vi "rrQA_Sub3.vi"(0 "U":dbl[](array[numeric]) format="%.2f", 2 "W":dbl[](array[numeric]) format="%.2f", 3 "T":dbl[](array[numeric]) format="%.2f") -> ()   [LabVIEW 2010]
uses:
  <vilib>/Utility/file.llb/Write To Spreadsheet File (DBL).vi
  <vilib>/Analysis/NI_AALBase.lvlib
panel:
  in  "u', w' data file":path
  out "Mean Time between events":dbl[](array[numeric])
  out "Loop Frame 1":i32
  out "Loop Frame 0":i32
  in  "LDA data?":bool
  in  "QA results file":path
  out "Quadrant shear totals":dbl[](array[numeric]) format="%.3f"
  out "% Time Spent in Quadrant":dbl[](array[numeric])
  out "u'w' (bar) total":dbl format="%.3f"
  in  "Threshold Array, H":dbl[](array[numeric])=[0.1] format="%.2f"
  out "XY Graph":cluster{dbl[], dbl[]}(graph)
  # "Quadrant Analysis Subroutine for Two-Component Velocity Data"
  # "Version 2.1 -RR"
  # "- FOR MANUAL ENTRY -"
  # "- ANALYSIS (OUTPUT) -"
  # "- FILE TO CREATE -"
  # "- THRESHOLD ARRAY -"
  # "- FOR PLUG-IN USE -"
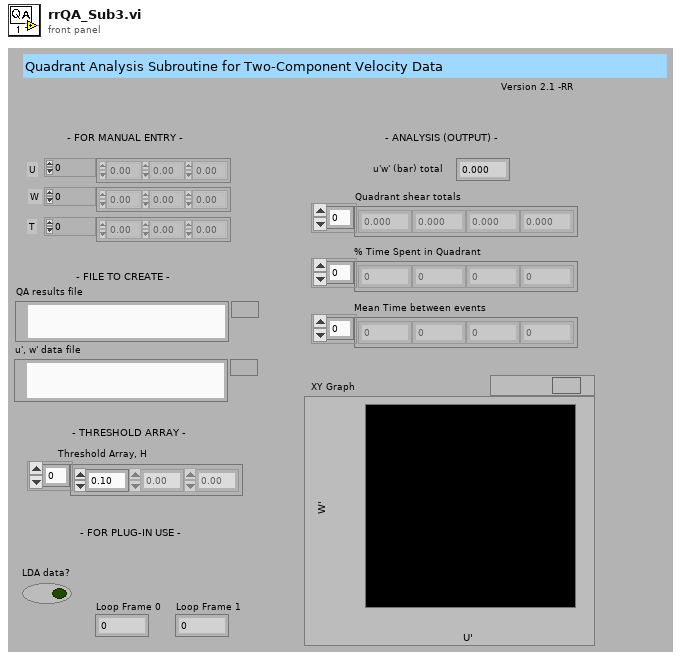
[diagram p1: front panel]
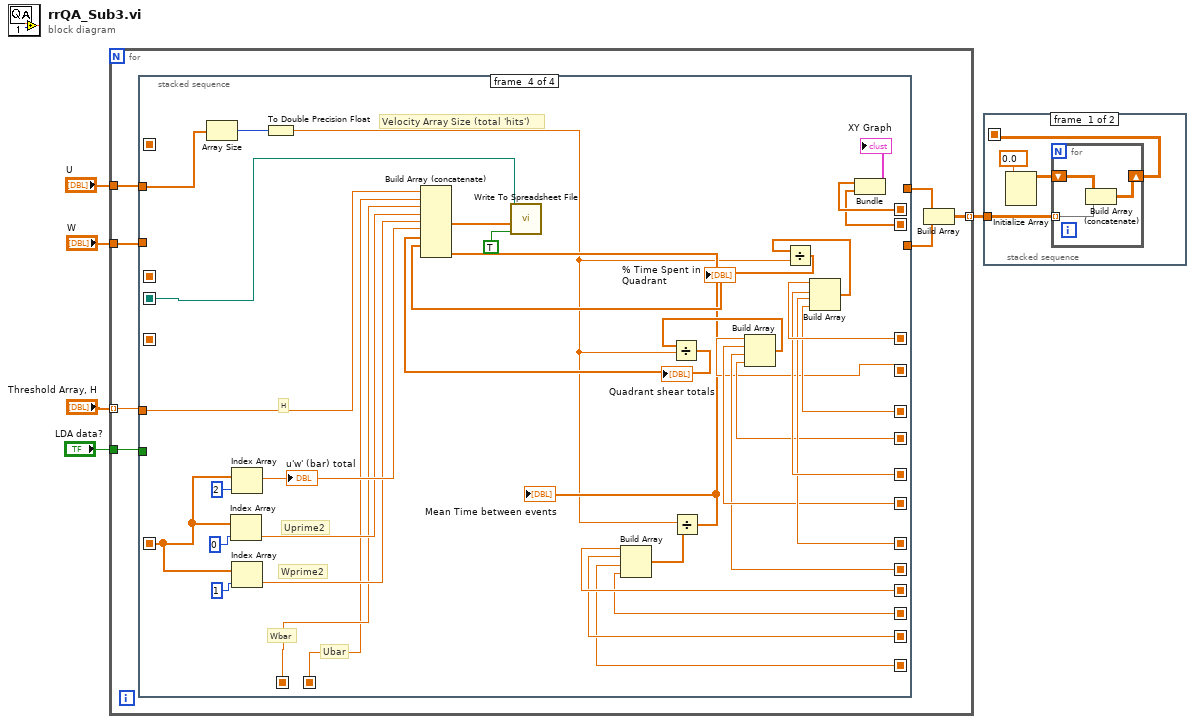
[diagram p0: block diagram]
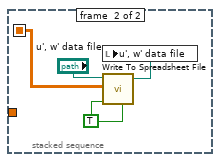
[diagram p2: hidden frame]
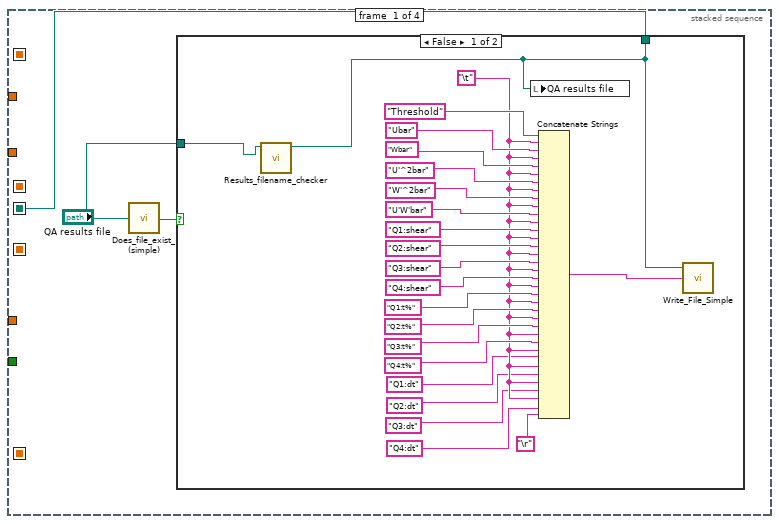
[diagram p3: hidden frame]
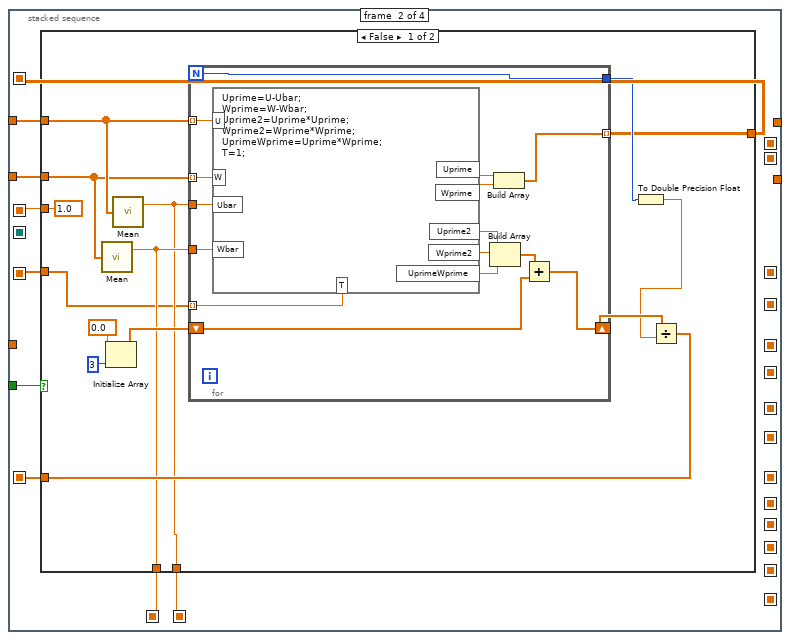
[diagram p5: hidden frame]
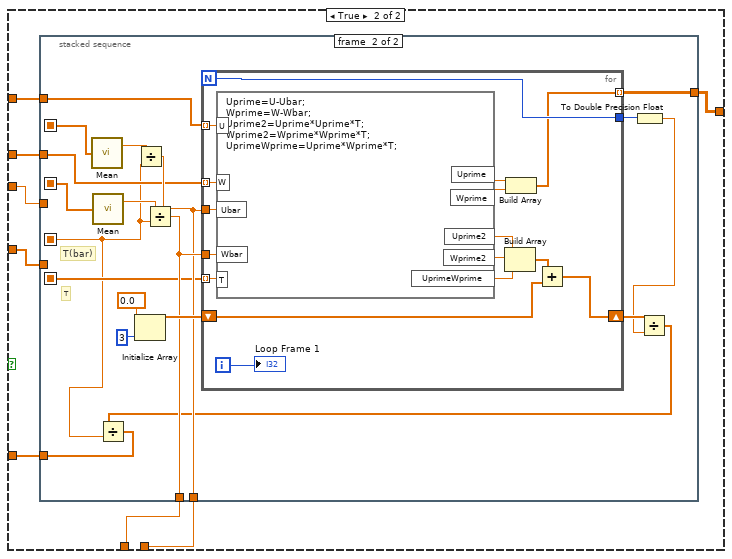
[diagram p6: hidden frame]
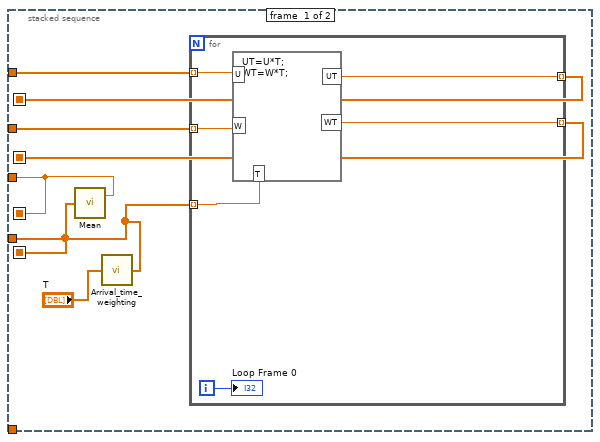
[diagram p7: hidden frame]
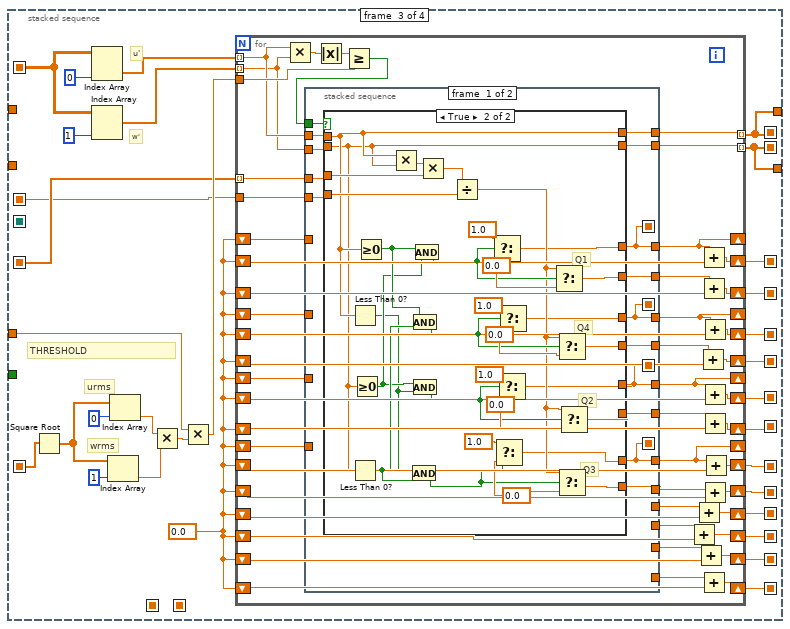
[diagram p8: hidden frame]
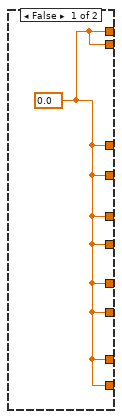
[diagram p9: hidden frame]
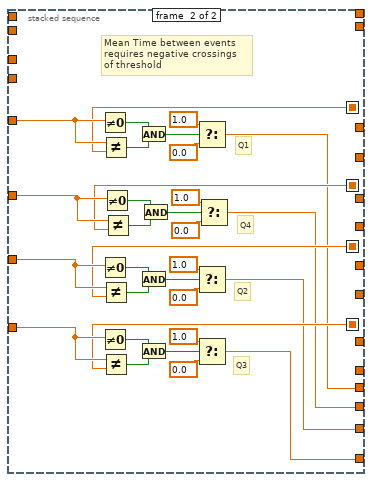
[diagram p10: hidden frame]
diagram:
  n1 = for {
    tunnel: "Threshold Array, H" -> [w12] mode=indexing
    tunnel: "U" -> [w11]
    tunnel: "W" -> [w10]
    tunnel: "LDA data?" -> [w9]
    tunnel: [w6] -> w1 mode=indexing
    n2 = stacked-sequence {
      seq-local: [_ w48 _ _] -> [_ _ w145 w319]
      seq-local: [_ _ w152 _] -> [_ _ _ w306]
      seq-local: [_ _ w153 _] -> [_ _ _ w329]
      seq-local: [_ _ w151 _] -> [_ _ _ w326]
      seq-local: [_ _ w150 _] -> [_ _ _ w322]
      seq-local: [_ _ w149 _] -> [_ _ _ w328]
      seq-local: [_ _ w148 _] -> [_ _ _ w324]
      seq-local: [_ _ w147 _] -> [_ _ _ w327]
      seq-local: [_ _ w146 _] -> [_ _ _ w323]
      seq-local: [_ w46 _ _] -> [_ _ _ w305]
      seq-local: [_ w45 _ _] -> [_ _ _ w304]
      seq-local: [_ w44 _ _] -> [_ _ w143 _]
      seq-local: [_ w43 _ _] -> [_ _ w144 _]
      seq-local: [_ w42 _ _] -> [_ _ w142 _]
      seq-local: [w15 _ _ _] -> [_ _ _ w314]
      seq-local: [_ _ w134 _] -> [_ _ _ w294]
      seq-local: [_ _ w135 _] -> [_ _ _ w295]
      seq-local: [_ _ w140 _] -> [_ _ _ w303]
      seq-local: [_ _ w139 _] -> [_ _ _ w302]
      seq-local: [_ _ w138 _] -> [_ _ _ w301]
      seq-local: [_ _ w137 _] -> [_ _ _ w300]
      tunnel: w9 -> [_ w47 _ _]
      tunnel: w11 -> [_ w41 _ w313]
      tunnel: w10 -> [_ w40 _ _]
      tunnel: w12 -> [_ _ w141 w296]
      tunnel: [_ _ w135 _] -> w8
      tunnel: [_ _ w134 _] -> w7
      frame #0 {
        n3 = call "Does_file_exist_(simple).vi"("Pathname"="QA results file") -> ("exists?"=w13:bool)
        n4 = case shown="False" w13 {
          tunnel: [w16 w39] -> w15
          tunnel: "QA results file" -> [w17 w39]
          frame False {
            w22 = "\t"
            n5 = call "Results_filename_checker.vi"("Results file"=w17) -> ("Results file output"=w16:path)  [unwired: 4 in, 3 out]
            n6 = local write "QA results file"(w16) -> ()
            n7 = Concatenate Strings("Threshold", w22, "Ubar", w22, "Wbar", w22, "U'^2bar", w22, "W'^2bar", w22, "U'W'bar", w22, "Q1:shear", w22, "Q2:shear", w22, "Q3:shear", w22, "Q4:shear", w22, "Q1:t%", w22, "Q2:t%", w22, "Q3:t%", w22, "Q4:t%", w22, "Q1:dt", w22, "Q2:dt", w22, "Q3:dt", w22, "Q4:dt", "\r") -> (w27:string)
            n8 = call "Write_File_Simple.vi"("character string"=w27, "file path"=w16) -> ()  [unwired: 1 in, 2 out]
          }
          frame True {
          }
        }
      }
      frame #1 {
        n9 = case shown="False" w47 {
          tunnel: [w58 w81] -> w48
          tunnel: w41 -> [w55 w85]
          tunnel: w40 -> [w54 w84]
          tunnel: [w53 w83] -> w46
          tunnel: [w52 w82] -> w45
          tunnel: [1.0 w80] -> w44
          tunnel: [w50 w79] -> w43
          tunnel: [w49 w78] -> w42
          frame False {
            n10 = call <vilib>:"Mean.vi"("X"=w54) -> ("mean"=w53:dbl)  [unwired: 1 out]
            n11 = Initialize Array(0.0, 3) -> (w61:dbl[])
            n12 = call <vilib>:"Mean.vi"("X"=w55) -> ("mean"=w52:dbl)  [unwired: 1 out]
            n13 = for {
              N -> [w68]
              tunnel: w55 -> [w77] mode=indexing
              tunnel: w54 -> [w76] mode=indexing
              shift-right: [w69] -> w59
              shift-left: w61 -> [w70]
              tunnel: [w68] -> w57
              tunnel: w52 -> [w66]
              tunnel: w53 -> [w65]
              tunnel: [w64] -> w50 mode=indexing
              tunnel: [w63] -> w49 mode=indexing
              n14 = formula code="Uprime=U-Ubar;\nWprime=W-Wbar;\nUprime2=Uprime*Uprime;\nWprime2=Wprime*Wprime;\nUprimeWprime=Uprime*Wprime;\nT=1;"("W"=w76, "U"=w77, "Ubar"=w66, "Wbar"=w65) -> ("Uprime"=w75:dbl, "Wprime"=w74:dbl, "Uprime2"=w73:dbl, "Wprime2"=w72:dbl, "UprimeWprime"=w67:dbl, "T"=w64:dbl)
              n15 = Build Array(w73, w72, w67) -> (w71:dbl[])
              n16 = Build Array(w75, w74) -> (w63:dbl[])
              n17 = Add(x=w71, y=w70) -> (x+y=w69:dbl[])
            }
            n18 = To Double Precision Float(number=w57) -> (double precision float=w56:dbl)
            n19 = Divide(x=w59, y=w56) -> (x/y=w58:dbl[])
          }
          frame True {
            n20 = stacked-sequence {
              seq-local: [w90 _] -> [_ w113]
              seq-local: [w89 _] -> [_ w114]
              seq-local: [w88 _] -> [_ w102]
              seq-local: [w86 _] -> [_ w106]
              tunnel: w85 -> [w92 w108]
              tunnel: w84 -> [w91 w107]
              tunnel: [_ w112] -> w83
              tunnel: [_ w109] -> w82
              tunnel: [_ w101] -> w81
              tunnel: [w88 _] -> w80
              tunnel: [w86 _] -> w79
              tunnel: [_ w99] -> w78
              frame #0 {
                n21 = call "Arrival_time_weighting.vi"("Arrival times"="T") -> ("Weighting"=w86:dbl[])
                n22 = call <vilib>:"Mean.vi"("X"=w86) -> ("mean"=w88:dbl)  [unwired: 1 out]
                n23 = for {
                  tunnel: w92 -> [w98] mode=indexing
                  tunnel: w91 -> [w97] mode=indexing
                  tunnel: w86 -> [w96] mode=indexing
                  tunnel: [w95] -> w90 mode=indexing
                  tunnel: [w94] -> w89 mode=indexing
                  i -> [w93]
                  n24 = formula code="UT=U*T;\nWT=W*T;"("T"=w96, "U"=w98, "W"=w97) -> ("UT"=w95:dbl, "WT"=w94:dbl)
                  "Loop Frame 0" <- w93
                }
              }
              frame #1 {
                # "T"
                # "T(bar)"
                n25 = call <vilib>:"Mean.vi"("X"=w113) -> ("mean"=w111:dbl)  [unwired: 1 out]
                n26 = call <vilib>:"Mean.vi"("X"=w114) -> ("mean"=w110:dbl)  [unwired: 1 out]
                n27 = Initialize Array(0.0, 3) -> (w115:dbl[])
                n28 = Divide(x=w111, y=w102) -> (x/y=w109:dbl)
                n29 = Divide(x=w110, y=w102) -> (x/y=w112:dbl)
                n30 = for {
                  N -> [w124]
                  tunnel: w108 -> [w133] mode=indexing
                  tunnel: w107 -> [w132] mode=indexing
                  shift-right: [w125] -> w104
                  shift-left: w115 -> [w126]
                  tunnel: [w124] -> w105
                  tunnel: w109 -> [w122]
                  tunnel: w112 -> [w121]
                  tunnel: w106 -> [w120] mode=indexing
                  tunnel: [w119] -> w99 mode=indexing
                  i -> [w118]
                  n31 = formula code="Uprime=U-Ubar;\nWprime=W-Wbar;\nUprime2=Uprime*Uprime*T;\nWprime2=Wprime*Wprime*T;\nUprimeWprime=Uprime*Wprime*T;"("W"=w132, "U"=w133, "Ubar"=w122, "Wbar"=w121, "T"=w120) -> ("Uprime"=w131:dbl, "Wprime"=w130:dbl, "Uprime2"=w129:dbl, "Wprime2"=w128:dbl, "UprimeWprime"=w123:dbl)
                  n32 = Build Array(w129, w128, w123) -> (w127:dbl[])
                  n33 = Build Array(w131, w130) -> (w119:dbl[])
                  n34 = Add(x=w127, y=w126) -> (x+y=w125:dbl[])
                  "Loop Frame 1" <- w118
                }
                n35 = To Double Precision Float(number=w105) -> (double precision float=w103:dbl)
                n36 = Divide(x=w104, y=w103) -> (x/y=w100:dbl[])
                n37 = Divide(x=w100, y=w102) -> (x/y=w101:dbl[])
              }
            }
          }
        }
      }
      frame #2 {
        w136 = 0.0
        # "THRESHOLD"
        # "wrms"
        # "urms"
        # "w'"
        # "u'"
        n38 = Square Root(x=w145) -> (sqrt(x)=w162:dbl[])
        n39 = Index Array(array=w142, index (col)=0) -> (element=w156:dbl[])  [unwired: 1 in]
        n40 = Index Array(array=w142, index (col)=1) -> (element=w155:dbl[])  [unwired: 1 in]
        n41 = Index Array(array=w162, index=1) -> (element=w158:dbl)
        n42 = Index Array(array=w162, index=0) -> (element=w159:dbl)
        n43 = Multiply(x=w159, y=w158) -> (x*y=w157:dbl)
        n44 = Multiply(x=w141, y=w157) -> (x*y=w154:dbl)
        n45 = for {
          tunnel: w156 -> [w202] mode=indexing
          tunnel: w155 -> [w201] mode=indexing
          tunnel: w154 -> [w212]
          tunnel: [w200] -> w135 mode=indexing
          tunnel: [w199] -> w134 mode=indexing
          shift-right: [w208] -> w152
          shift-left: w136 -> [w191]
          shift-right: [w211] -> w150
          shift-left: w136 -> [w189]
          shift-right: [w210] -> w148
          shift-left: w136 -> [w187]
          shift-right: [w209] -> w146
          shift-left: w136 -> [w185]
          shift-right: [w204] -> w153
          shift-left: w136 -> [w192]
          shift-right: [w207] -> w151
          shift-left: w136 -> [w190]
          shift-right: [w206] -> w149
          shift-left: w136 -> [w188]
          shift-right: [w205] -> w147
          shift-left: w136 -> [w186]
          tunnel: w144 -> [w198] mode=indexing
          tunnel: w143 -> [w197]
          shift-right: [w184] -> _
          shift-left: w136 -> [w180]
          shift-right: [w183] -> _
          shift-left: w136 -> [w177]
          shift-right: [w182] -> _
          shift-left: w136 -> [w178]
          shift-right: [w181] -> _
          shift-left: w136 -> [w179]
          shift-right: [w172] -> w140
          shift-left: w136 -> [w168]
          shift-right: [w171] -> w139
          shift-left: w136 -> [w167]
          shift-right: [w170] -> w138
          shift-left: w136 -> [w166]
          shift-right: [w169] -> w137
          shift-left: w136 -> [w165]
          n46 = Multiply(x=w202, y=w201) -> (x*y=w214:dbl)
          n47 = Absolute Value(x=w214) -> (abs(x)=w213:dbl)
          n48 = Greater Or Equal?(x=w213, y=w212) -> (x >= y?=w203:bool)
          n49 = stacked-sequence {
            seq-local: [w218 _] -> [_ w269]
            seq-local: [w217 _] -> [_ w268]
            seq-local: [w216 _] -> [_ w267]
            seq-local: [w215 _] -> [_ w266]
            tunnel: w203 -> [w229 _]
            tunnel: w202 -> [w228 _]
            tunnel: w201 -> [w227 _]
            tunnel: [w226 _] -> w200
            tunnel: [w225 _] -> w199
            tunnel: w198 -> [w224 _]
            tunnel: w197 -> [w223 _]
            tunnel: [w218 _] -> w184
            tunnel: [w222 _] -> w196
            tunnel: [w217 _] -> w183
            tunnel: [w221 _] -> w195
            tunnel: [w216 _] -> w182
            tunnel: [w220 _] -> w194
            tunnel: [w215 _] -> w181
            tunnel: [w219 _] -> w193
            tunnel: w180 -> [_ w270]
            tunnel: w179 -> [_ w273]
            tunnel: w178 -> [_ w272]
            tunnel: w177 -> [_ w271]
            tunnel: [_ w265] -> w176
            tunnel: [_ w264] -> w175
            tunnel: [_ w263] -> w174
            tunnel: [_ w262] -> w173
            frame #0 {
              n50 = case shown="True" w229 {
                tunnel: w228 -> [_ w238]
                tunnel: w227 -> [_ w237]
                tunnel: [w230 w238] -> w226
                tunnel: [w230 w237] -> w225
                tunnel: [w230 w245] -> w222
                tunnel: [w230 w244] -> w221
                tunnel: [w230 w243] -> w220
                tunnel: [w230 w242] -> w219
                tunnel: [w230 w234] -> w218
                tunnel: [w230 w233] -> w217
                tunnel: [w230 w232] -> w216
                tunnel: [w230 w231] -> w215
                tunnel: w224 -> [_ w239]
                tunnel: w223 -> [_ w241]
                frame False {
                  w230 = 0.0
                }
                frame True {
                  w258 = 0.0
                  w259 = 0.0
                  w260 = 0.0
                  w261 = 0.0
                  # "Q3"
                  # "Q2"
                  # "Q4"
                  # "Q1"
                  n51 = Less Than 0?(x=w238) -> (x < 0?=w250:bool)
                  n52 = Less Than 0?(x=w237) -> (x < 0?=w252:bool)
                  n53 = Greater Or Equal To 0?(x=w237) -> (x >= 0?=w251:bool)
                  n54 = Greater Or Equal To 0?(x=w238) -> (x >= 0?=w253:bool)
                  n55 = Multiply(x=w238, y=w237) -> (x*y=w236:dbl)
                  n56 = And(x=w250, y=w252) -> (x .and. y?=w246:bool)
                  n57 = And(x=w253, y=w252) -> (x .and. y?=w248:bool)
                  n58 = And(x=w251, y=w250) -> (x .and. y?=w247:bool)
                  n59 = And(x=w253, y=w251) -> (x .and. y?=w249:bool)
                  n60 = Multiply(x=w236, y=w239) -> (x*y=w235:dbl)
                  n61 = Divide(x=w235, y=w241) -> (x/y=w240:dbl)
                  n62 = Select(t=1.0, s=w249, f=w261) -> (s? t:f=w234:dbl)
                  n63 = Select(t=1.0, s=w246, f=w258) -> (s? t:f=w231:dbl)
                  n64 = Select(t=1.0, s=w247, f=w259) -> (s? t:f=w232:dbl)
                  n65 = Select(t=1.0, s=w248, f=w260) -> (s? t:f=w233:dbl)
                  n66 = Select(t=w240, s=w249, f=w261) -> (s? t:f=w245:dbl)
                  n67 = Select(t=w240, s=w248, f=w260) -> (s? t:f=w244:dbl)
                  n68 = Select(t=w240, s=w246, f=w258) -> (s? t:f=w242:dbl)
                  n69 = Select(t=w240, s=w247, f=w259) -> (s? t:f=w243:dbl)
                }
              }
            }
            frame #1 {
              # "Q3"
              # "Q2"
              # "Q4"
              # "Q1"
              # "Mean Time between events\nrequires negative crossings\nof threshold"
              n70 = Not Equal To 0?(x=w270) -> (x != 0?=w292:bool)
              n71 = Not Equal To 0?(x=w272) -> (x != 0?=w282:bool)
              n72 = Not Equal To 0?(x=w273) -> (x != 0?=w275:bool)
              n73 = Not Equal?(x=w270, y=w269) -> (x != y?=w293:bool)
              n74 = Not Equal?(x=w272, y=w267) -> (x != y?=w283:bool)
              n75 = Not Equal?(x=w273, y=w266) -> (x != y?=w274:bool)
              n76 = Not Equal To 0?(x=w271) -> (x != 0?=w285:bool)
              n77 = Not Equal?(x=w271, y=w268) -> (x != y?=w284:bool)
              n78 = And(x=w292, y=w293) -> (x .and. y?=w289:bool)
              n79 = And(x=w282, y=w283) -> (x .and. y?=w279:bool)
              n80 = And(x=w275, y=w274) -> (x .and. y?=w278:bool)
              n81 = And(x=w285, y=w284) -> (x .and. y?=w288:bool)
              n82 = Select(t=1.0, s=w289, f=0.0) -> (s? t:f=w265:dbl)
              n83 = Select(t=1.0, s=w279, f=0.0) -> (s? t:f=w263:dbl)
              n84 = Select(t=1.0, s=w278, f=0.0) -> (s? t:f=w262:dbl)
              n85 = Select(t=1.0, s=w288, f=0.0) -> (s? t:f=w264:dbl)
            }
          }
          n86 = Add(x=w175, y=w167) -> (x+y=w171:dbl)
          n87 = Add(x=w176, y=w168) -> (x+y=w172:dbl)
          n88 = Add(x=w174, y=w166) -> (x+y=w170:dbl)
          n89 = Add(x=w195, y=w189) -> (x+y=w211:dbl)
          n90 = Add(x=w184, y=w192) -> (x+y=w204:dbl)
          n91 = Add(x=w196, y=w191) -> (x+y=w208:dbl)
          n92 = Add(x=w173, y=w165) -> (x+y=w169:dbl)
          n93 = Add(x=w183, y=w190) -> (x+y=w207:dbl)
          n94 = Add(x=w182, y=w188) -> (x+y=w206:dbl)
          n95 = Add(x=w194, y=w187) -> (x+y=w210:dbl)
          n96 = Add(x=w193, y=w185) -> (x+y=w209:dbl)
          n97 = Add(x=w181, y=w186) -> (x+y=w205:dbl)
        }
      }
      frame #3 {
        # "Velocity Array Size (total 'hits')"
        # "Wprime2"
        # "Uprime2"
        # "H"
        # "Wbar"
        # "Ubar"
        n98 = Array Size(array=w313) -> (size(s)=w310:i32)
        n99 = Index Array(array=w319, index=0) -> (element=w318:dbl)
        n100 = Index Array(array=w319, index=2) -> (element=w325:dbl)
        "u'w' (bar) total" <- w325
        n101 = Index Array(array=w319, index=1) -> (element=w317:dbl)
        n102 = To Double Precision Float(number=w310) -> (double precision float=w297:dbl)
        n103 = Build Array(w303, w301, w300, w302) -> (w298:dbl[])
        n104 = Divide(x=w297, y=w298) -> (x/y=w299:dbl[])
        "Mean Time between events" <- w299
        n105 = Build Array(w306, w324, w323, w322) -> (w312:dbl[])
        n106 = Divide(x=w312, y=w297) -> (x/y=w311:dbl[])
        "Quadrant shear totals" <- w311
        n107 = Build Array(w329, w328, w327, w326) -> (w308:dbl[])
        n108 = Divide(x=w308, y=w297) -> (x/y=w309:dbl[])
        "% Time Spent in Quadrant" <- w309
        n109 = Build Array (concatenate)(w296, w304, w305, w318, w317, w325, w311, w309, w299) -> (w315:dbl[])
        n110 = call-poly <vilib>:"Write To Spreadsheet File.vi"("append to file? (new file:F)"=TRUE, "1D data"=w315, "file path (dialog if empty)"=w314) -> ()  [unwired: 3 in, 3 out]
        n111 = Bundle(w295, w294) -> (→"XY Graph":cluster{dbl[], dbl[]})  [unwired: 1 out]
      }
    }
    n112 = Build Array(w8, w7) -> (w6:dbl[][])
  }
  n113 = stacked-sequence {
    seq-local: [w333 _] -> [_ w338]
    tunnel: w1 -> [w334 _]
    frame #0 {
      n114 = Initialize Array(0.0) -> (w331:dbl[][])  [unwired: 2 out]
      n115 = for {
        shift-right: [w335] -> w333
        shift-left: w331 -> [w336]
        tunnel: w334 -> [w337] mode=indexing
        n116 = Build Array (concatenate)(w336, w337) -> (w335:dbl[][])
      }
    }
    frame #1 {
      w341 = TRUE
      n117 = call-poly <vilib>:"Write To Spreadsheet File.vi"("transpose? (no:F)"=w341, "append to file? (new file:F)"=w341, "2D data"=w338, "file path (dialog if empty)"="u', w' data file") -> ("new file path (Not A Path if cancelled)"=w340:path)  [unwired: 2 in, 2 out]
      n118 = local write "u', w' data file"(w340) -> ()
    }
  }
